vi "Disc_Test.vi"(1 "LT_Pressed":bool, 2 "RB_Pressed":bool) -> ()   [LabVIEW 2018]
uses:
  Subsytems/Intake_Disc/Intake_Disc_Notifier.ctl
  Subsytems/Intake_Disc/Intake_Disc_Control_Type.ctl
  <vilib>/Rock Robotics/WPI/Solenoid/WPI_SolenoidValue.ctl
  <vilib>/Rock Robotics/WPI/DriverStation/WPI_DriverStationRobotMode2.ctl
  Global_Variables/Intake_Disc_Globals.vi
  Global_Variables/Robot_Global_Data.vi
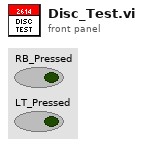
[diagram p1: front panel]
types:
  T1 = typedef "WPI_DriverStationRobotMode2.ctl" = enum16{"Autonomous Disabled", "Autonomous Enabled", "Teleop Disabled", "Teleop Enabled", "Disconnected", "Finish", "Test Disabled", "Test Enabled", "Emergency Stopped"}
  T2 = typedef "Intake_Disc_Notifier.ctl" = cluster{"Intake_Disc_Control_Type":T3, "Manual_Disc_Toggle":bool, "Disc_Toggle":bool, "Disc_Toggle_State":bool, "Manual_Press_Toggle":bool, "Disc_Press_State":bool, "Press_Toggle":bool, "Press_Pnuematic":T4, "Disc_Pnuematic":T4, "Disc_Notifier":refnum<notifier>, "Step":i32}
  T3 = typedef "Intake_Disc_Control_Type.ctl" = enum16{"No_Op", "Manual_Disc_Toggle", "Disc_Toggle", "Manual_Press_Toggle", "Press_Toggle", "Acquire_Hatch", "Retract"}
  T4 = typedef "WPI_SolenoidValue.ctl" = enum16{"Off", "On", "Forward", "Reverse"}
  T5 = typedef "WPI_SolenoidDevRef.ctl" = cluster{"DevStatus":errorcluster, "Pneumatics Control Module":u8, "Forward Solenoid Channel":T6, "Reverse Solenoid Channel":T6}
  T6 = typedef "WPI_SolenoidChannel.ctl" = enum8{"Solenoid 0", "Solenoid 1", "Solenoid 2", "Solenoid 3", "Solenoid 4", "Solenoid 5", "Solenoid 6", "Solenoid 7", "Invalid"}
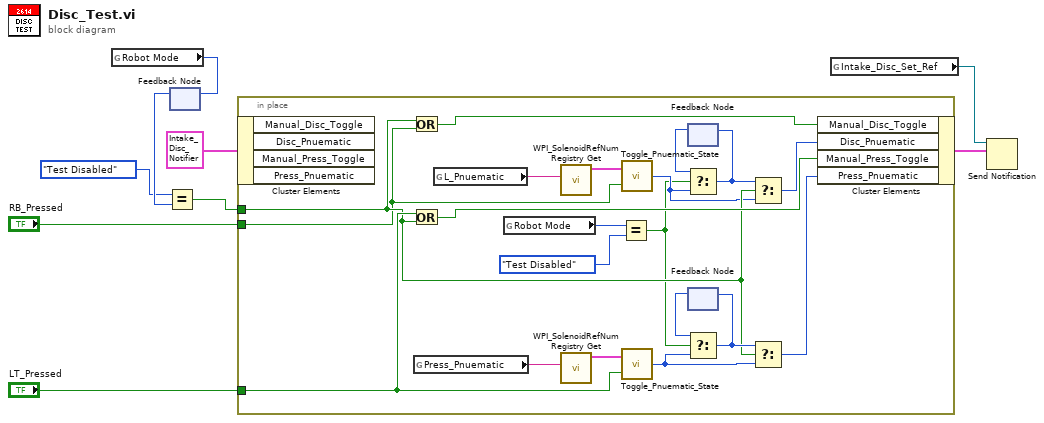
[diagram p0: block diagram]
diagram:
  n1 = global read "Robot_Global_Data.vi" "Robot Mode"() -> (w4:T1)
  n2 = feedback-in #1(w4) -> ()
  n3 = feedback #1() -> (w3:T1)  [unwired: 1 in]
  n4 = Equal?(x=WPI_DriverStationRobotMode2."Test Disabled", y=w3) -> (x = y?=w1:bool)
  n5 = in-place {
    in-place-border: "RB_Pressed" -> [w15]
    in-place-border: "LT_Pressed" -> [w29]
    in-place-border: w1 -> [w16]
    n6 = in-place-cluster #2(T2 {"Intake_Disc_Control_Type"=enum."No_Op", "Manual_Disc_Toggle"=FALSE, "Disc_Toggle"=FALSE, "Disc_Toggle_State"=FALSE, "Manual_Press_Toggle"=FALSE, "Disc_Press_State"=FALSE, "Press_Toggle"=FALSE, "Press_Pnuematic"=enum."Forward", "Disc_Pnuematic"=enum."Forward", "Disc_Notifier"=refnum, "Step"=0} ("Intake_Disc_Notifier")) -> ()  [unwired: 4 out]
    n7 = Or(x=w16, y=w15) -> (x .or. y?=w19:bool)
    n8 = Or(x=w29, y=w16) -> (x .or. y?=w26:bool)
    n9 = global read "Intake_Disc_Globals.vi" "Press_Pnuematic"() -> (w27:string)
    n10 = global read "Intake_Disc_Globals.vi" "L_Pnuematic"() -> (w18:string)
    n11 = global read "Robot_Global_Data.vi" "Robot Mode"() -> (w24:T1)
    n12 = call <vilib>:"WPI_SolenoidRefNum Registry Get.vi"("refnum name"=w18) -> ("SolenoidDevRef"=w17:T5)  [unwired: 9 in, 1 out]
    n13 = call <vilib>:"WPI_SolenoidRefNum Registry Get.vi"("refnum name"=w27) -> ("SolenoidDevRef"=w28:T5)  [unwired: 9 in, 1 out]
    n14 = Equal?(x=w24, y=WPI_DriverStationRobotMode2."Test Disabled") -> (x = y?=w10:bool)
    n15 = call "Toggle_Pnuematic_State.vi"("Boolean"=w15, "Solonoid_In"=w17) -> ("Solenoid_Out"=w12:T4)
    n16 = call "Toggle_Pnuematic_State.vi"("Boolean"=w29, "Solonoid_In"=w28) -> ("Solenoid_Out"=w22:T4)
    n17 = feedback #3() -> (w11:T4)  [unwired: 1 in]
    n18 = Select(t=w11, s=w10, f=w12) -> (s? t:f=w13:T4)
    n19 = feedback-in #3(w13) -> ()
    n20 = feedback #4() -> (w21:T4)  [unwired: 1 in]
    n21 = Select(t=w21, s=w10, f=w22) -> (s? t:f=w20:T4)
    n22 = feedback-in #4(w20) -> ()
    n23 = Select(t=w13, s=w16, f=w12) -> (s? t:f=w14:T4)
    n24 = Select(t=w20, s=w16, f=w22) -> (s? t:f=w25:T4)
    n25 = in-place-cluster #2("Manual_Disc_Toggle"=w19, "Disc_Pnuematic"=w14, "Manual_Press_Toggle"=w26, "Press_Pnuematic"=w25) -> (w9:T2)
  }
  n26 = global read "Intake_Disc_Globals.vi" "Intake_Disc_Set_Ref"() -> (w8:refnum<notifier>)
  n27 = Send Notification(notification=w9, notifier=w8) -> ()  [unwired: 1 in, 2 out]
